vi "ATICalbMatrix.vi"(11 "Automation Refnum in":refnum<k7>) -> (0 "CalbArray":dbl[](array[numeric]), 3 "CalbMatrix":dbl[][](array[numeric]))   [LabVIEW 2024]
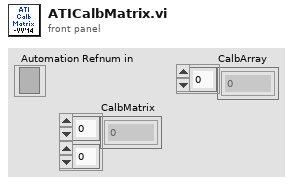
[diagram p1: front panel]
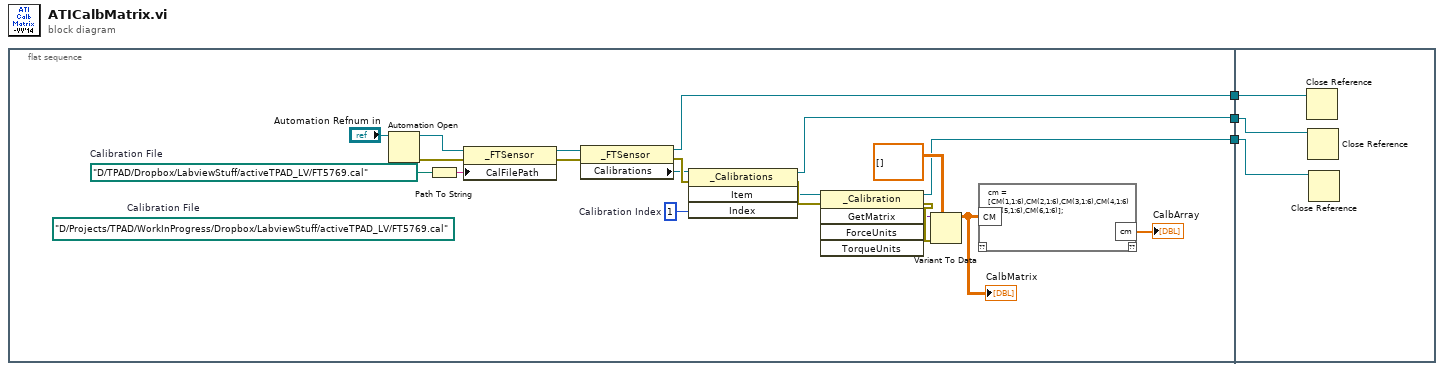
[diagram p0: block diagram]
diagram:
  n1 = flat-sequence {
    tunnel: [w6] -> w3
    tunnel: [w5] -> w2
    tunnel: [w4] -> w1
    tunnel: w3 -> [w26]
    tunnel: w2 -> [w24]
    tunnel: w1 -> [w25]
    frame #0 {
      w23 = i16 1  # Calibration Index
      w21 = path "D:/TPAD/Dropbox/LabviewStuff/activeTPAD_LV/FT5769.cal"  # Calibration File
      (unwired) path "D:/Projects/TPAD/WorkInProgress/Dropbox/LabviewStuff/activeTPAD_LV/FT5769.cal"  # Calibration File
      n2 = Automation Open(Automation Refnum="Automation Refnum in") -> (Automation Refnum=w8:refnum<k7>, error out=w16:errorcluster)  [unwired: 3 in]
      n3 = Path To String(path=w21) -> (string=w9:string)
      n4 = property class="_FTSensor"(reference=w8, error in=w16, "CalFilePath"=w9) -> (reference out=w10:refnum<k7>, error out=w17:errorcluster)
      n5 = property class="_FTSensor"(reference=w10, error in=w17) -> (reference out=w6:refnum<k7>, error out=w18:errorcluster, "Calibrations"=w11:refnum<k7>)
      n6 = invoke class="_Calibrations" method="Item"(reference=w11, error in=w18, "Index"=w23) -> (reference out=w5:refnum<k7>, error out=w19:errorcluster, "Item"=w12:refnum<k7>)  [unwired: 1 in, 1 out]
      n7 = invoke class="_Calibration" method="GetMatrix"(reference=w12, error in=w19) -> (reference out=w4:refnum<k7>, error out=w20:errorcluster, "GetMatrix"=w14:variant)  [unwired: 3 in, 2 out]
      n8 = Variant To Data(error in=w20, type=dbl[][] [], Variant=w14) -> (data=w15:dbl[][])  [unwired: 1 out]
      "CalbMatrix" <- w15
      n9 = mathscript code="cm = [CM(1,1:6),CM(2,1:6),CM(3,1:6),CM(4,1:6),CM(5,1:6),CM(6,1:6)];"("CM"=w15) -> ("cm"=→"CalbArray":dbl[])  [unwired: 1 in, 1 out]
    }
    frame #1 {
      n10 = Close Reference(reference=w26) -> ()  [unwired: 1 in, 1 out]
      n11 = Close Reference(reference=w24) -> ()  [unwired: 1 in, 1 out]
      n12 = Close Reference(reference=w25) -> ()  [unwired: 1 in, 1 out]
    }
  }
